vi "OpenVIReference.vi"(5 "VI Path To Open":path=path "Z:/Tests/3.0/FlexLVAdapter/Refnums/VIRefnum/VIToRun.vi") -> (0 "error out":errorcluster, 2 "VI Refnum":refnum<vi>)   [LabVIEW 2011]
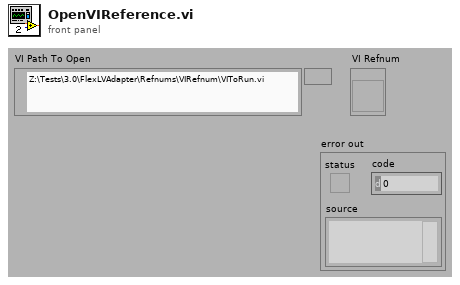
[diagram p1: front panel]
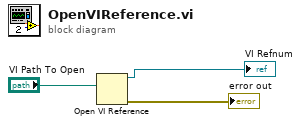
[diagram p0: block diagram]
diagram:
  n1 = Open VI Reference(vi path="VI Path To Open") -> (vi reference=→"VI Refnum":refnum<vi>, error out=→"error out":errorcluster)  [unwired: 1 in, 4 out]
